vi "Button_event.vi"() -> ()   [LabVIEW 2017]
panel:
  out "Waveform Chart":dbl(graph)
  in  "stop":bool
  in  "OK button":bool
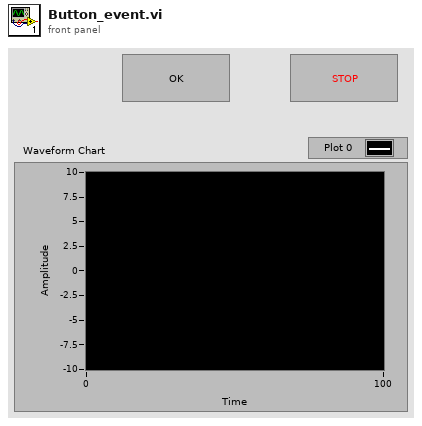
[diagram p1: front panel]
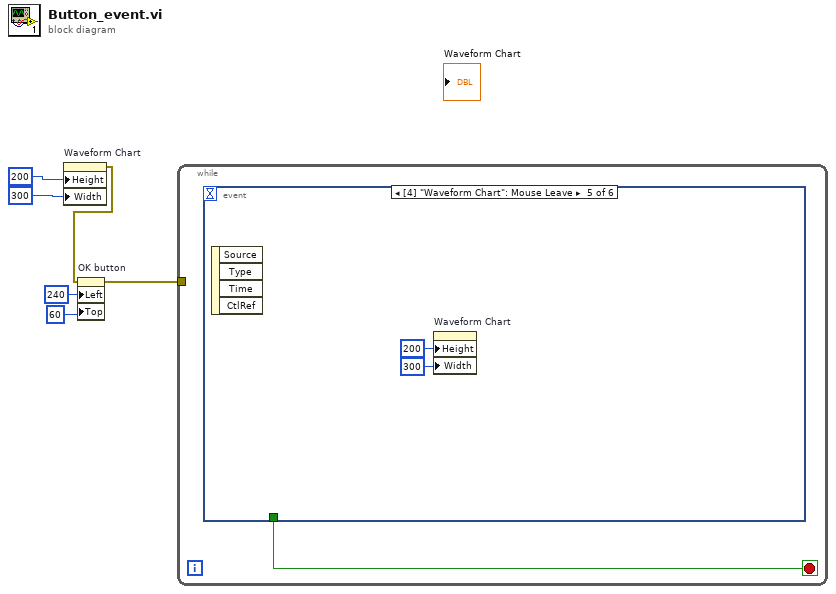
[diagram p0: block diagram]
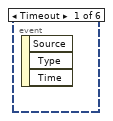
[diagram p2: hidden frame]
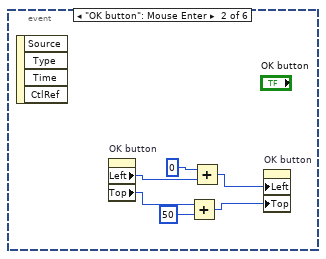
[diagram p3: hidden frame]
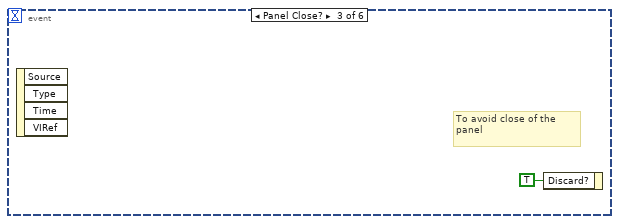
[diagram p4: hidden frame]
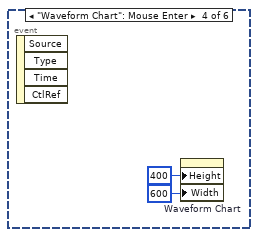
[diagram p5: hidden frame]
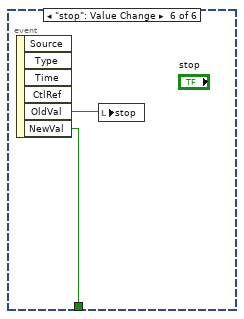
[diagram p6: hidden frame]
diagram:
  n1 = property on="Waveform Chart" class="WFChart (strict)"("Height"=u32 200 ("Plot Area:Size:Height"), "Width"=u32 300 ("Plot Area:Size:Width")) -> (error out=w1:errorcluster)  [unwired: 2 in, 1 out]
  n2 = property on="OK button" class="Bool"(error in=w1, "Left"=240 ("Position:Left"), "Top"=60 ("Position:Top")) -> (error out=w6:errorcluster)  [unwired: 1 in, 1 out]
  n3 = while {
    tunnel: w6 -> [_]
    stop <- w7 stop-if-true
    n4 = event shown="[4] \"Waveform Chart\": Mouse Leave" {
      selector: _ -> [_ _ _ _ _ _]
      dyn-events: _ -> [_ _ _ _ _ _]
      timeout: _ -> [_ _ _ _ _ _]
      tunnel: [_ _ _ _ _ w19] -> w7
      event Timeout {
        n5 = event-data() -> ()  [unwired: 1 in, 3 out]
      }
      event "OK button": Mouse Enter {
        n6 = event-data() -> ()  [unwired: 1 in, 4 out]
        n7 = property on="OK button" class="Bool"() -> ("Left"=w13:i32, "Top"=w12:i32)  [unwired: 2 in, 2 out]
        n8 = Add(x=w12, y=50) -> (x+y=w8:i32)
        n9 = Add(x=0, y=w13) -> (x+y=w9:i32)
        n10 = property on="OK button" class="Bool"("Left"=w9, "Top"=w8) -> ()  [unwired: 2 in, 2 out]
      }
      event Panel Close? {
        # "To avoid close of the\npanel"
        n11 = event-data() -> ()  [unwired: 1 in, 4 out]
        n12 = event-data("Discard?"=TRUE) -> ()  [unwired: 1 in, 1 out]
      }
      event "Waveform Chart": Mouse Enter {
        n13 = event-data() -> ()  [unwired: 1 in, 4 out]
        n14 = property on="Waveform Chart" class="WFChart (strict)"("Height"=u32 400 ("Plot Area:Size:Height"), "Width"=u32 600 ("Plot Area:Size:Width")) -> ()  [unwired: 2 in, 2 out]
      }
      event "Waveform Chart": Mouse Leave {
        n15 = event-data() -> ()  [unwired: 1 in, 4 out]
        n16 = property on="Waveform Chart" class="WFChart (strict)"("Height"=u32 200 ("Plot Area:Size:Height"), "Width"=u32 300 ("Plot Area:Size:Width")) -> ()  [unwired: 2 in, 2 out]
      }
      event "stop": Value Change {
        n17 = event-data() -> ("OldVal"=w20:bool, "NewVal"=w19:bool)  [unwired: 1 in, 4 out]
        n18 = local write "stop"(w20) -> ()
      }
    }
  }
